vi "Client Template.vi"() -> ()   [LabVIEW 2025, in "OOB gRPC Client.lvlib"]
uses:
  OOB gRPC Client.lvlib
  RPC Messages/hwval_BoolRequest.ctl
  RPC Messages/hwval_ExportRequest.ctl
panel:
  in  "stop":bool
  in  "Export":bool
  in  "Export File Type":string(combo)="RAW"
  in  "PauseResume":bool caption="Pause"
  out "OOB gRPC Port":i32
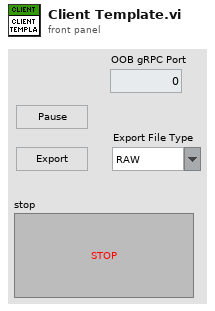
[diagram p1: front panel]
types:
  T1 = typedef "OOB gRPC Client.lvlib/hwval_BoolRequest.ctl" = cluster{"BooleanData":bool}
  T2 = typedef "OOB gRPC Client.lvlib/hwval_ExportRequest.ctl" = cluster{"FileType":string}
  T3 = typedef "grpc-lvsupport-release.lvlib/grpcId.ctl" = u64
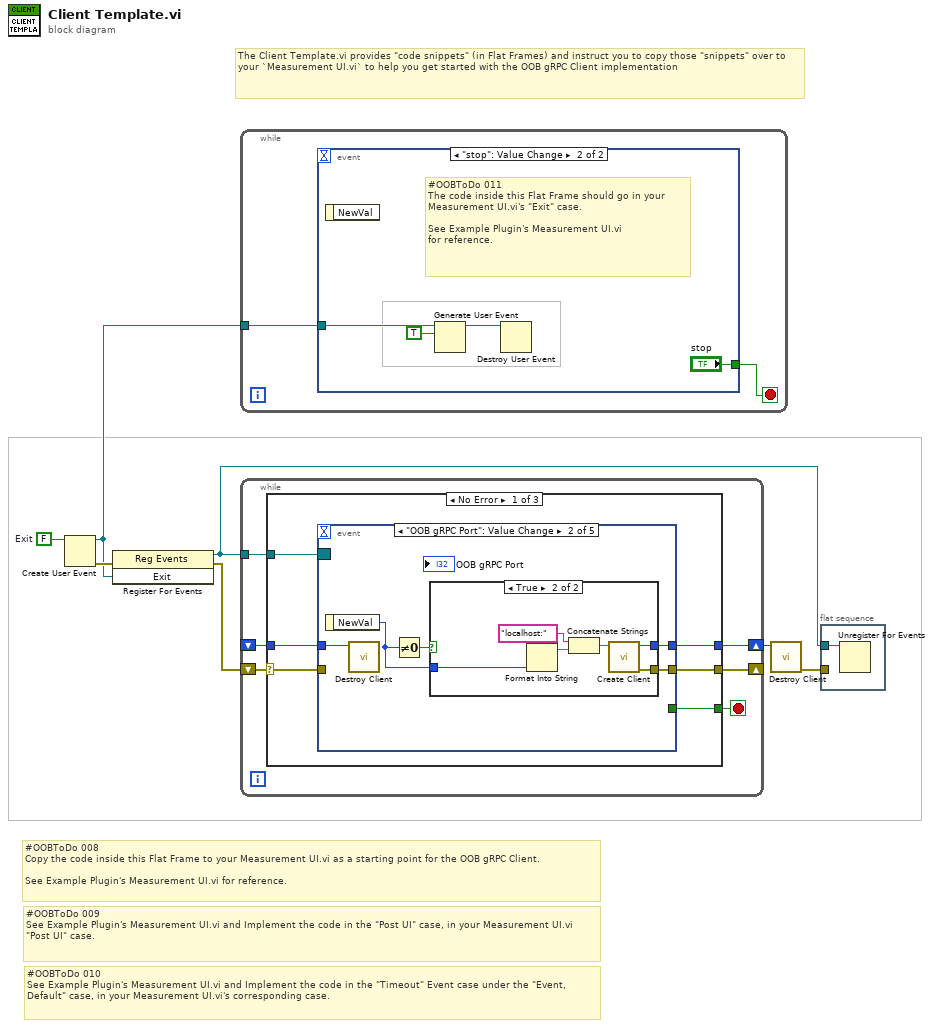
[diagram p0: block diagram]
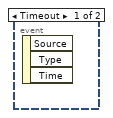
[diagram p2: hidden frame]
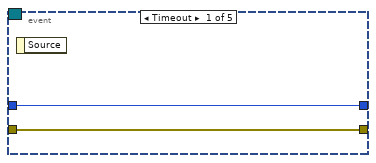
[diagram p3: hidden frame]
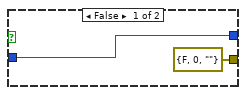
[diagram p4: hidden frame]
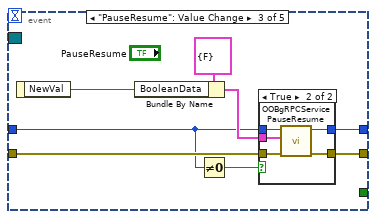
[diagram p5: hidden frame]
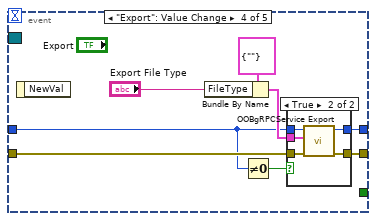
[diagram p7: hidden frame]
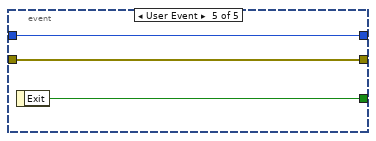
[diagram p9: hidden frame]
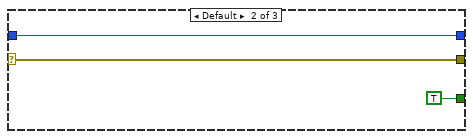
[diagram p10: hidden frame]
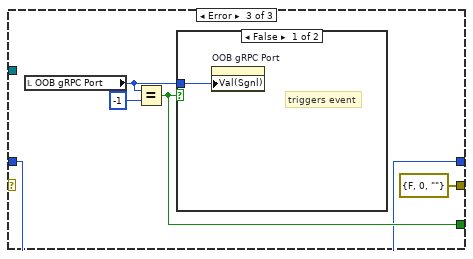
[diagram p11: hidden frame]
diagram:
  w7 = FALSE  # Exit
  # "The Client Template.vi provides \"code snippets\" (in Flat Frames) and instruct you to copy those \"snippets\" over to your `Measurement UI.vi` to help you get started with the OOB gRPC Client implementation"
  # "#OOBToDo 010 \nSee Example Plugin's Measurement UI.vi and Implement the code in the \"Timeout\" Event case under the \"Event, Default\" case, in your Measurement UI.vi's corresponding case."
  # "#OOBToDo 009 \nSee Example Plugin's Measurement UI.vi and Implement the code in the \"Post UI\" case, in your Measurement UI.vi \"Post UI\" case."
  # "#OOBToDo 008\nCopy the code inside this Flat Frame to your Measurement UI.vi as a starting point for the OOB gRPC Client.\n\nSee Example Plugin's Measurement UI.vi for reference."
  n1 = Create User Event(user event datatype=w7) -> (user event=w1:refnum<user-event>, error out=w6:errorcluster)  [unwired: 1 in]
  n2 = register-events(error in=w6, w1) -> (reference out=w2:refnum<event-registration>, error out=w5:errorcluster)  [unwired: 1 in]
  n3 = while {
    tunnel: w1 -> [w8]
    stop <- w9 stop-if-true
    n4 = event shown="[1] \"stop\": Value Change" {
      selector: _ -> [_ _]
      dyn-events: _ -> [_ _]
      timeout: _ -> [_ _]
      tunnel: [_ "stop"] -> w9
      tunnel: w8 -> [_ w10]
      event Timeout {
        n5 = event-data() -> ()  [unwired: 1 in, 3 out]
      }
      event "stop": Value Change {
        # "#OOBToDo 011\nThe code inside this Flat Frame should go in your Measurement UI.vi's \"Exit\" case.\n\nSee Example Plugin's Measurement UI.vi for reference."
        n6 = event-data() -> ()  [unwired: 1 in, 1 out]
        n7 = Generate User Event(user event=w10, event data cluster=TRUE ("event data")) -> (user event out=w11:refnum<user-event>)  [unwired: 2 in, 1 out]
        n8 = Destroy User Event(user event=w11) -> ()  [unwired: 1 in, 1 out]
      }
    }
  }
  n9 = while {
    tunnel: w2 -> [w16]
    shift-right: [w17] -> _
    shift-left: w5 -> [w19]
    shift-right: [w14] -> w3
    shift-left: _ -> [w15]
    stop <- w18 stop-if-true
    n10 = case shown="No Error" w19 {
      selector: w19 -> [w23 w74 _]
      tunnel: [w20 TRUE w79] -> w18
      tunnel: [w24 w74 errorcluster {"status"=FALSE, "code"=0, "source"=""} ("error IO")] -> w17
      tunnel: w16 -> [w25 _ _]
      tunnel: w15 -> [w22 w75 w78]
      tunnel: [w21 w75 w78] -> w14
      frame No Error {
        n11 = event shown="[1] \"OOB gRPC Port\": Value Change" {
          selector: w25 -> [_ _ _ _ _]
          dyn-events: _ -> [_ _ _ _ _]
          timeout: _ -> [_ _ _ _ _]
          tunnel: [w27 w32 w47 w62 w71] -> w24
          tunnel: w23 -> [w27 _ w46 w61 w71]
          tunnel: w22 -> [w26 w31 w41 w57 w72]
          tunnel: [w26 w30 w48 w63 w72] -> w21
          tunnel: [_ _ _ _ w73] -> w20
          event Timeout {
            n12 = event-data() -> ()  [unwired: 1 in, 1 out]
          }
          event "OOB gRPC Port": Value Change {
            n13 = event-data() -> ("NewVal"=w28:i32)  [unwired: 1 in]
            n14 = call "Destroy Client.vi"("gRPC ID"=w31) -> ()  [unwired: 10 in, 1 out]
            n15 = Not Equal To 0?(x=w28) -> (x != 0?=w29:bool)
            n16 = case shown="True" w29 {
              tunnel: [errorcluster {"status"=FALSE, "code"=0, "source"=""} ("error out") w40] -> w32
              tunnel: w28 -> [w34 w36]
              tunnel: [w34 w35] -> w30
              frame False {
              }
              frame True {
                n17 = Format Into String(w36) -> (resulting string=w39:string)  [unwired: 3 in, 1 out]
                n18 = Concatenate Strings("localhost:" ("string"), w39) -> (w37:string)
                n19 = call "Create Client.vi"("address"=w37) -> ("error out"=w40:errorcluster, "gRPC ID Out"=w35:T3)  [unwired: 9 in]
              }
            }
          }
          event "PauseResume": Value Change {
            n20 = event-data() -> ("NewVal"=w43:bool)  [unwired: 1 in]
            n21 = Bundle By Name(cluster=T1 {"BooleanData"=FALSE} ("Request Data"), "BooleanData"=w43) -> (w44:T1)
            n22 = Not Equal To 0?(x=w41) -> (x != 0?=w42:bool)
            n23 = case shown="True" w42 {
              tunnel: [w50 w55] -> w48
              tunnel: [w49 w54] -> w47
              tunnel: w41 -> [w50 w53]
              tunnel: w46 -> [w49 w52]
              tunnel: w44 -> [_ w51]
              frame False {
              }
              frame True {
                n24 = call "OOBgRPCService PauseResume.vi"("error in"=w52, "Request Data"=w51, "gRPC ID"=w53) -> ("error out"=w54:errorcluster, "gRPC ID out"=w55:T3)  [unwired: 6 in, 1 out]
              }
            }
          }
          event "Export": Value Change {
            n25 = event-data() -> ()  [unwired: 1 in, 1 out]
            n26 = Bundle By Name(cluster=T2 {"FileType"=""} ("Request Data"), "FileType"="Export File Type") -> (w59:T2)
            n27 = Not Equal To 0?(x=w57) -> (x != 0?=w58:bool)
            n28 = case shown="True" w58 {
              tunnel: [w65 w70] -> w63
              tunnel: [w64 w69] -> w62
              tunnel: w57 -> [w65 w68]
              tunnel: w61 -> [w64 w67]
              tunnel: w59 -> [_ w66]
              frame False {
              }
              frame True {
                n29 = call "OOBgRPCService Export.vi"("error in"=w67, "Request Data"=w66, "gRPC ID"=w68) -> ("error out"=w69:errorcluster, "gRPC ID out"=w70:T3)  [unwired: 6 in, 1 out]
              }
            }
          }
          event User Event {
            n30 = event-data() -> ("Exit"=w73:bool)  [unwired: 1 in]
          }
        }
      }
      frame Default {
      }
      frame Error {
        n31 = local read "OOB gRPC Port"() -> (w81:i32)
        n32 = Equal?(x=w81, y=-1 ("x")) -> (x = y?=w79:bool)
        n33 = case shown="False" w79 {
          tunnel: w81 -> [w82 _]
          frame False {
            # "triggers event"
            n34 = property on="OOB gRPC Port" class="DigNum (strict)"("Val(Sgnl)"=w82) -> ()  [unwired: 2 in, 2 out]
          }
          frame True {
          }
        }
      }
    }
  }
  n35 = call "Destroy Client.vi"("gRPC ID"=w3) -> ("error out"=w4:errorcluster)  [unwired: 10 in]
  n36 = flat-sequence {
    tunnel: w2 -> [w83]
    tunnel: w4 -> [_]
    frame #0 {
      n37 = Unregister For Events(event registration refnum=w83) -> ()  [unwired: 1 in, 1 out]
    }
  }
